vi "Helper SubVI - Linear Quantization.vi"(10 "bits":i32=1 min=1 max=64, 11 "signal":dbl[](array[numeric])) -> (3 "quantized signal":dbl[](array[numeric]))   [LabVIEW 2023]
doc: "Quantizes the wavelet packet coefficients."
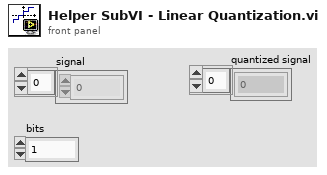
[diagram p1: front panel]
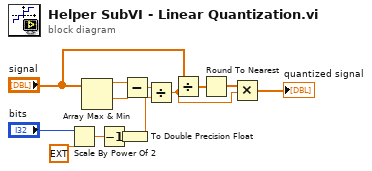
[diagram p0: block diagram]
diagram:
  n1 = Scale By Power Of 2(n="bits", x=ext 1.0) -> (x*2^n=w11:ext)
  n2 = Array Max & Min(array="signal") -> (max value=w1:dbl, min value=w2:dbl)  [unwired: 2 out]
  n3 = Decrement(x=w11) -> (x-1=w12:ext)
  n4 = To Double Precision Float(number=w12) -> (double precision float=w13:dbl)
  n5 = Subtract(x=w1, y=w2) -> (x-y=w3:dbl)
  n6 = Divide(x=w3, y=w13) -> (x/y=w6:dbl)
  n7 = Divide(x="signal", y=w6) -> (x/y=w4:dbl[])
  n8 = Round To Nearest(number=w4) -> (nearest integer value=w5:dbl[])
  n9 = Multiply(x=w5, y=w6) -> (x*y=→"quantized signal":dbl[])
